vi "Check.vi"(8 "error in (no error)":errorcluster, 9 "Type":string, 10 "Wafer ID":string, 11 "EpiWrapper in":refnum<class "EpiWrapper.lvclass">) -> (0 "error out":errorcluster, 1 "Tested?":bool, 2 "Exists?":bool, 3 "EpiWrapper out":refnum<class "EpiWrapper.lvclass">)   [LabVIEW 2012, in "EpiWrapper.lvclass"]
uses:
  EpiWrapper.lvclass
  EpiWrapper.lvclass/EpiWrapper.ctl
  LotData.lvclass
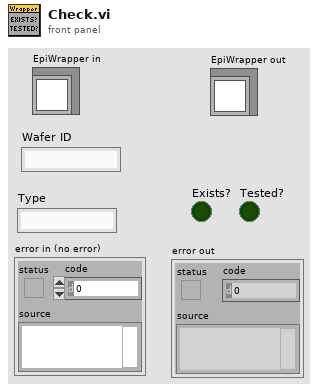
[diagram p1: front panel]
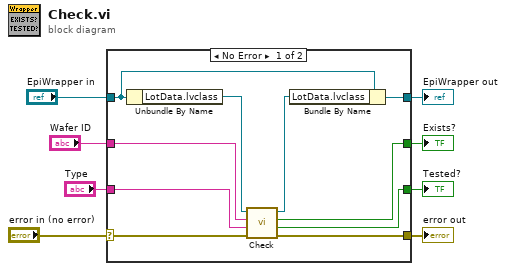
[diagram p0: block diagram]
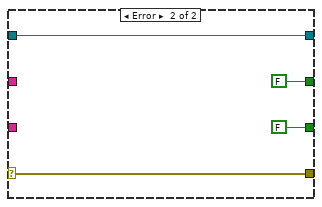
[diagram p2: hidden frame]
diagram:
  n1 = case shown="No Error" "error in (no error)" {
    selector: "error in (no error)" -> [w15 w22]
    tunnel: [w9 w22] -> w7
    tunnel: [w10 w21] -> w5
    tunnel: "EpiWrapper in" -> [w12 w21]
    tunnel: "Wafer ID" -> [w17 _]
    tunnel: "Type" -> [w16 _]
    tunnel: [w14 FALSE ("Exists?")] -> w2
    tunnel: [w13 FALSE ("Tested?")] -> w1
    frame No Error {
      n2 = Unbundle By Name(w12) -> ("LotData.lvclass"=w18:refnum<class "LotData.lvclass">)
      n3 = call "Check.vi"("error in (no error)"=w15, "Type"=w16, "Wafer ID"=w17, "LotData in"=w18) -> ("error out"=w9:errorcluster, "Tested?"=w13:bool, "Exists?"=w14:bool, "LotData out"=w11:refnum<class "LotData.lvclass">)
      n4 = Bundle By Name(cluster=w12, "LotData.lvclass"=w11) -> (w10:refnum<class "EpiWrapper.lvclass">)
    }
    frame Error {
    }
  }
  "error out" <- w7
  "EpiWrapper out" <- w5
  "Exists?" <- w2
  "Tested?" <- w1
